vi "Optiscan_Device.vi"(7 "Device-specific in":variant, 8 "error in (no error)":errorcluster, 10 "Position in":dbl[](array[numeric]), 11 "Operation":T2(ring)) -> (0 "error out":errorcluster, 1 "Device properties":cluster{"Axes":string[], "Tolerance":dbl[][]}, 2 "Position out":dbl[](array[numeric]), 3 "Status":T1, 5 "Device-specific out":variant)   [LabVIEW 2018]
uses:
  <vilib>/Instr/_visa.llb/VISA Open Access Mode.ctl
  <vilib>/Instr/_visa.llb/VISA Configure Serial Port (Instr).vi
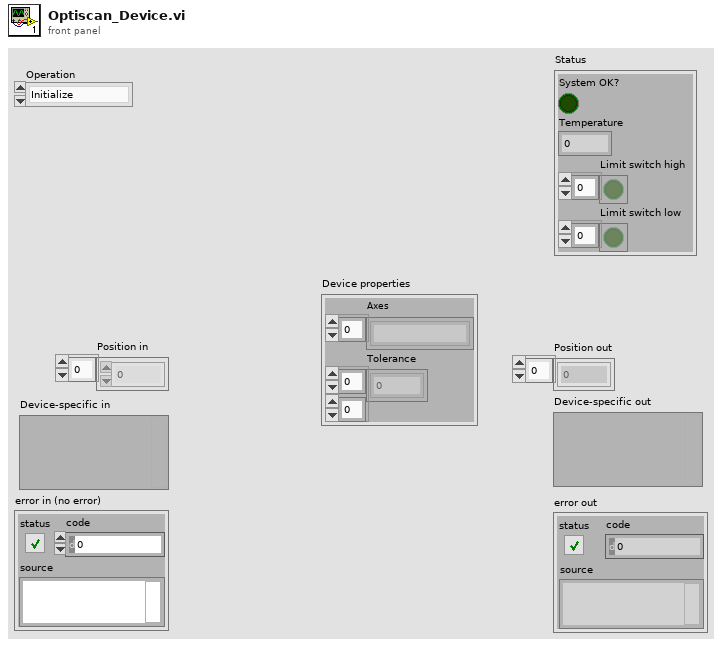
[diagram p1: front panel]
types:
  T1 = cluster{"System OK?":bool, "Temperature":dbl, "Limit switch high":bool[], "Limit switch low":bool[]}
  T2 = enum16{"Initialize", "Shut down", "Set position", "Get position", "Get status", "Other settings"}
  T3 = cluster{"COM port":refnum<visa-resource-name>, "Timeout":u32}
  T4 = typedef "VISA Open Access Mode.ctl" = u32
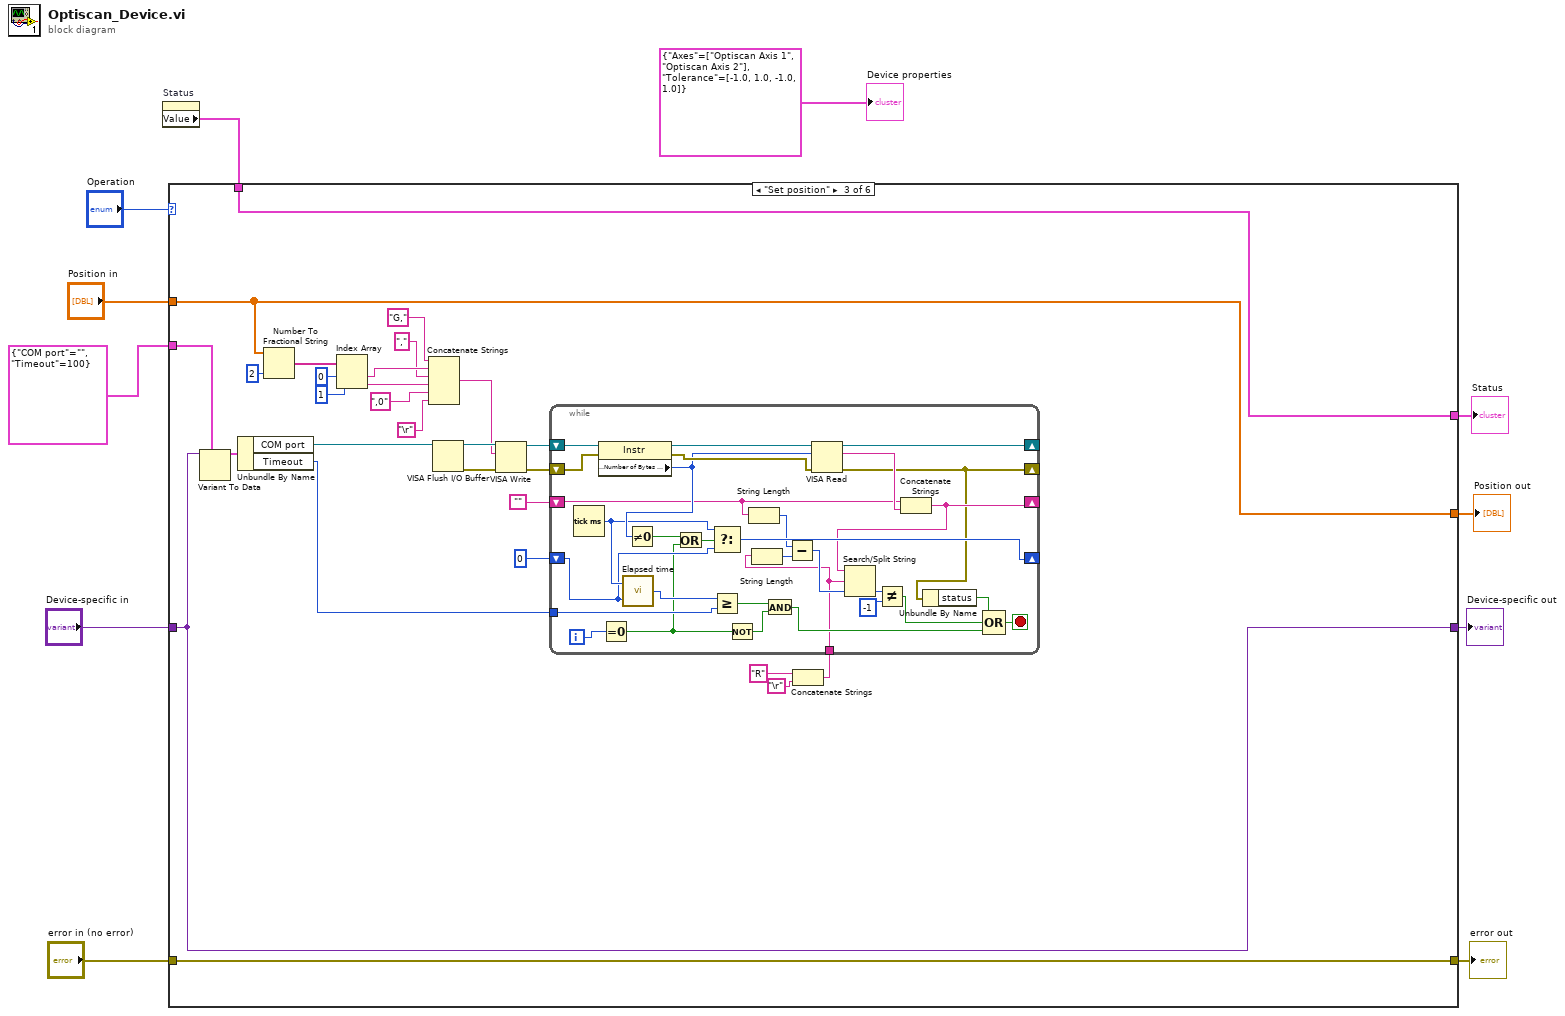
[diagram p0: block diagram]
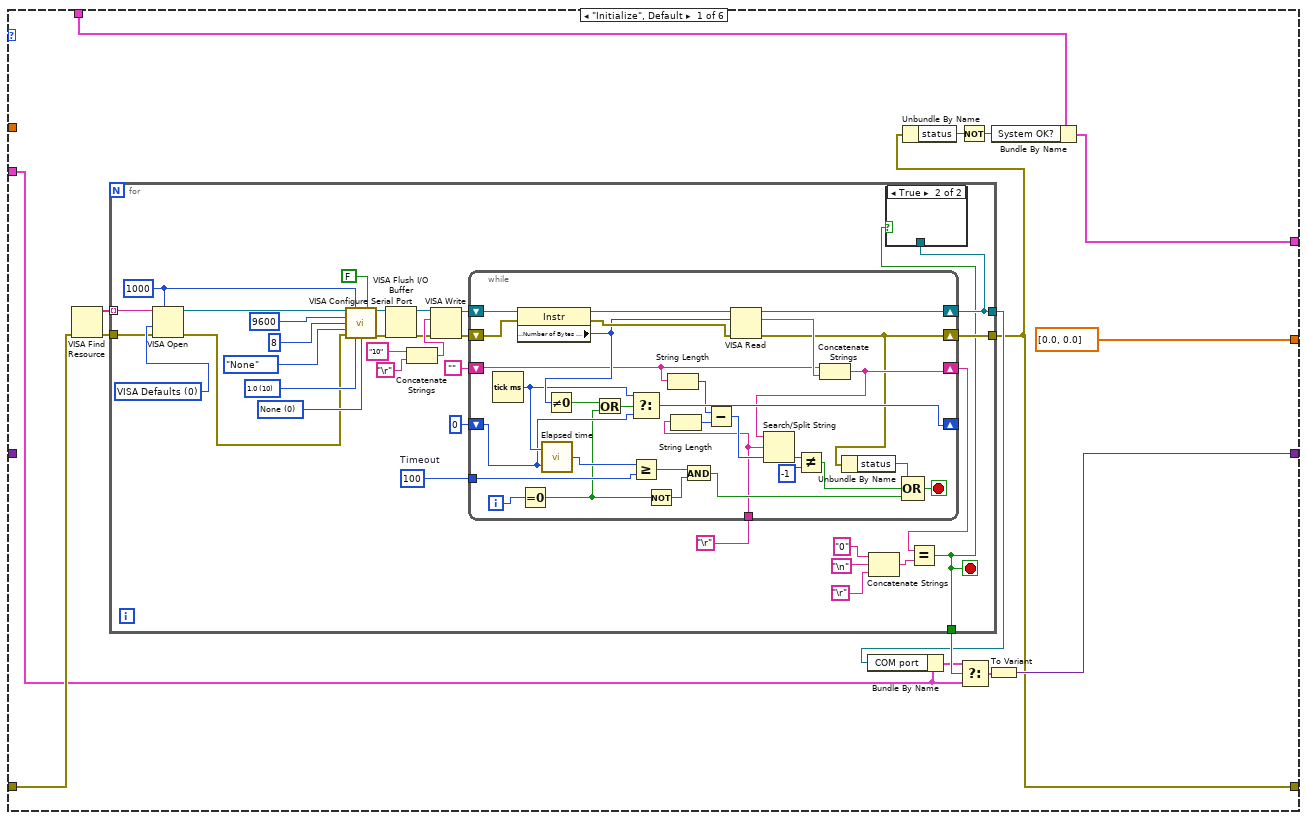
[diagram p2: hidden frame]
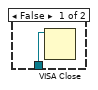
[diagram p3: hidden frame]
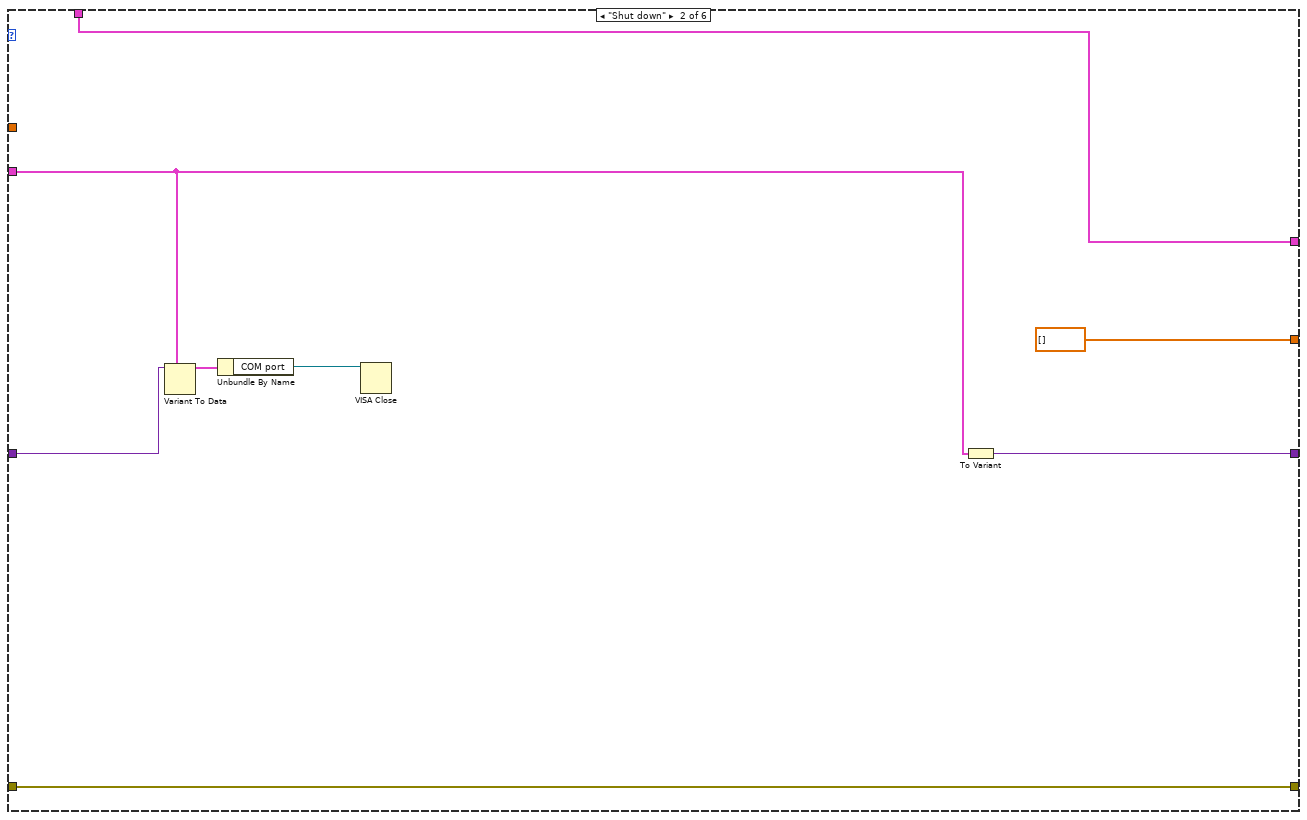
[diagram p4: hidden frame]
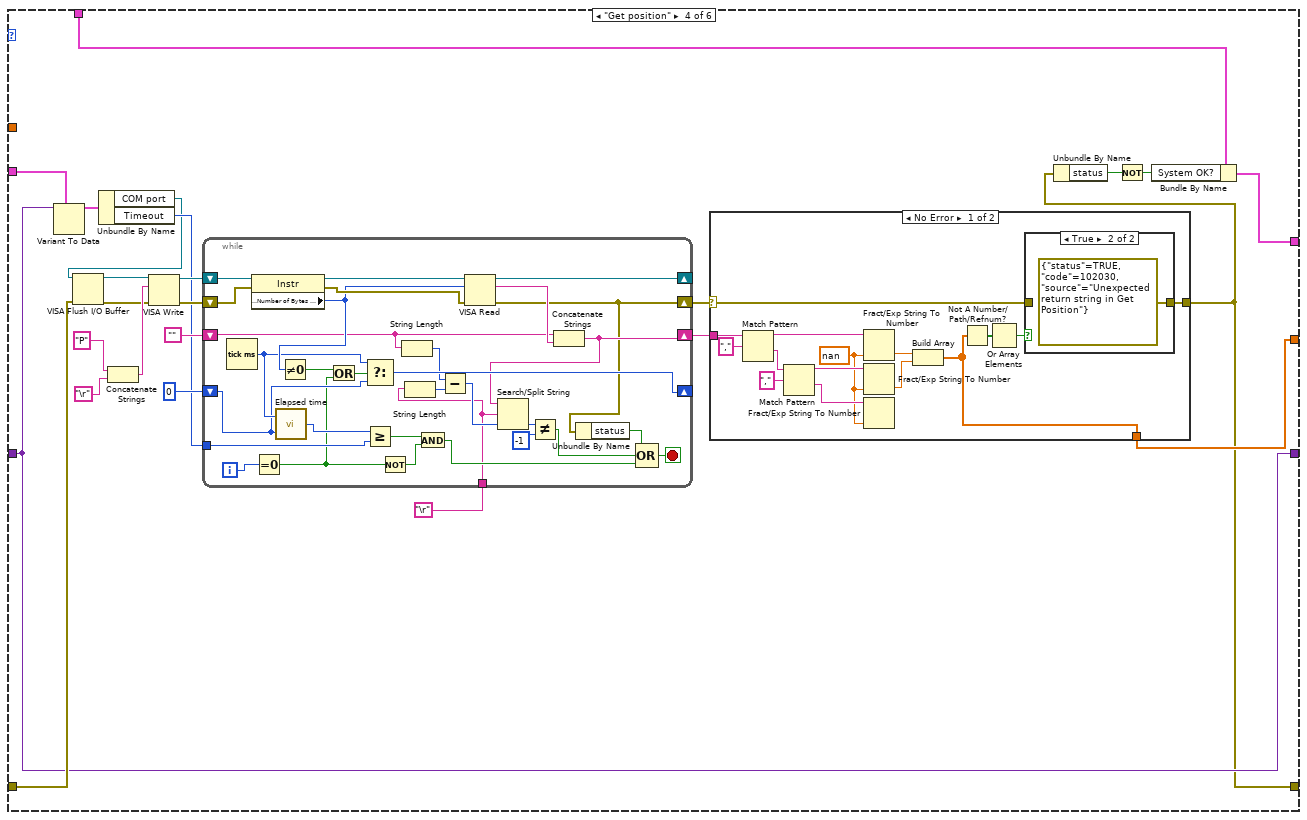
[diagram p5: hidden frame]
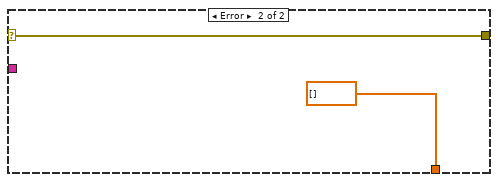
[diagram p7: hidden frame]
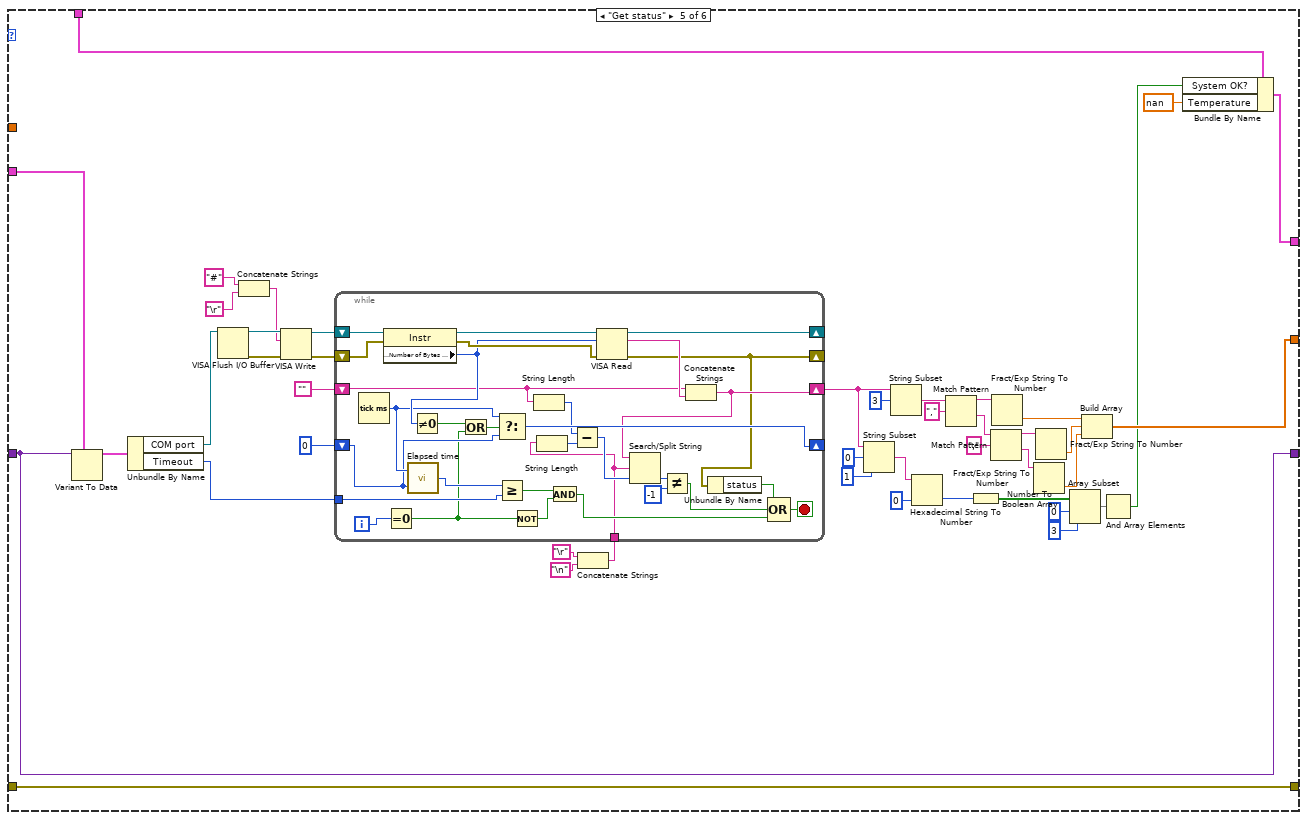
[diagram p8: hidden frame]
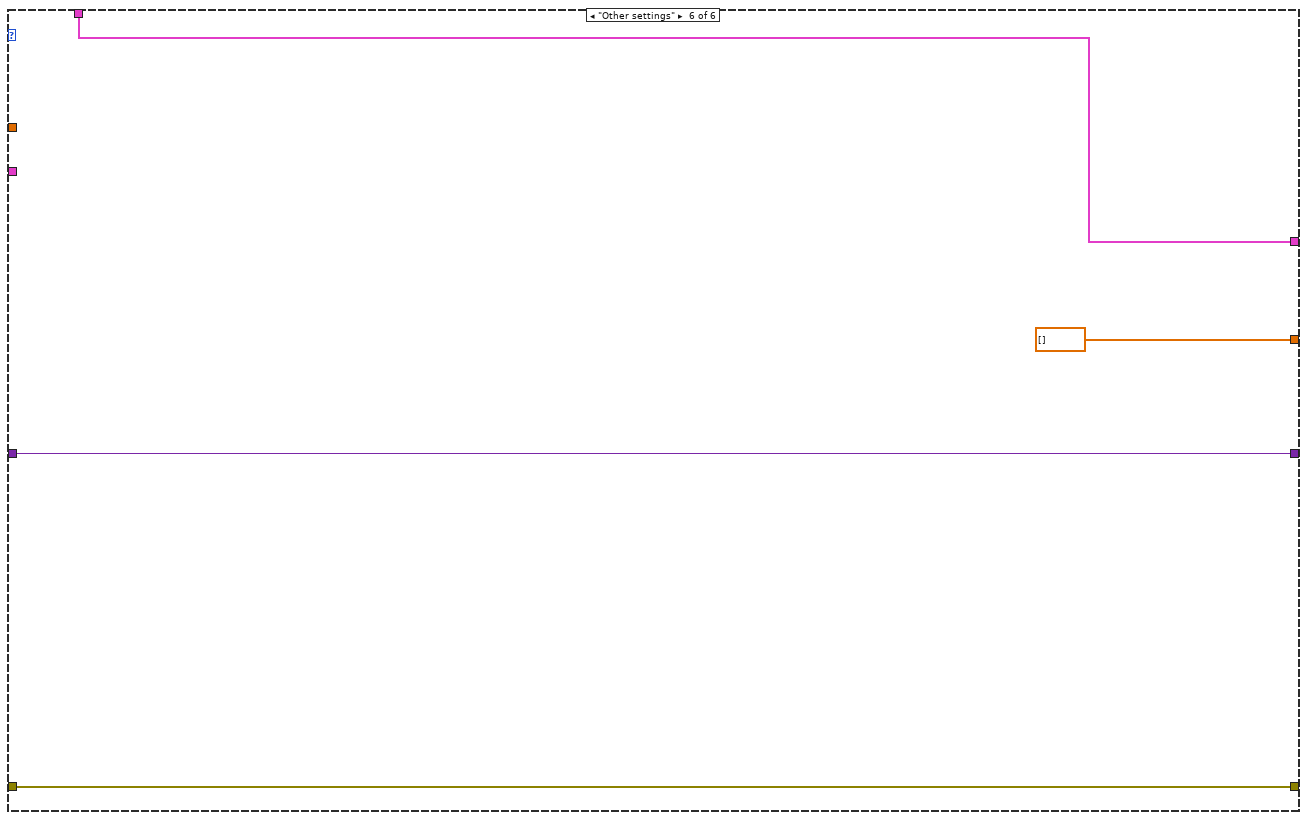
[diagram p9: hidden frame]
diagram:
  n1 = property on="Status" class="Clust (strict)"() -> ("Value"=w10:T1)  [unwired: 2 in, 2 out]
  n2 = case shown="\"Set position\"" "Operation" {
    tunnel: "Position in" -> [_ _ w101 _ _ _]
    tunnel: w10 -> [w26 w99 w127 w163 w276 w311]
    tunnel: [w25 w99 w127 w162 w275 w311] -> w9
    tunnel: "Device-specific in" -> [_ w96 w117 w170 w261 w310]
    tunnel: [dbl[] [0.0, 0.0] ("Position in") dbl[] [] ("Position in") w101 w164 w235 dbl[] [] ("Position in")] -> w6
    tunnel: [w18 w93 w117 w170 w261 w310] -> w5
    tunnel: [w15 w98 w126 w161 w273 w309] -> w4
    tunnel: "error in (no error)" -> [w16 w98 w126 w171 w273 w309]
    tunnel: T3 {"COM port"="", "Timeout"=100} -> [w13 w94 w116 w169 w260 _]
    frame "Initialize", Default {
      n3 = VISA Find Resource(8:w16) -> (0:w17:errorcluster, 3:w23:string[])  [unwired: 2 in, 1 out]
      n4 = for {
        tunnel: w23 -> [w49] mode=indexing
        tunnel: [w34] -> w21
        tunnel: [w28] -> w22
        tunnel: w17 -> [w36]
        tunnel: [w35] -> w15
        stop <- w28 stop-if-true
        w39 = u32 100  # Timeout
        w50 = u32 1000 ("timeout (10sec)")
        w52 = T4 0 items=["VISA Defaults"=0, "Exclusive Lock"=1, "Load Configured Settings"=4] ("Access Mode")
        w54 = u16 0 items=["None", "XON/XOFF", "RTS/CTS", "XON/XOFF & RTS/CTS", "DTR/DSR", "XON/XOFF & DTR/DSR"] ("flow control (0:none)")
        w55 = u16 10 items=["1.0"=10, "1.5"=15, "2.0"=20] ("stop bits (10: 1 bit)")
        n5 = VISA Open(timeout (0)=w50, access mode=w52, error in (no error)=w36, VISA resource name=w49) -> (VISA resource name=w53:refnum<visa-resource-name>, error out=w51:errorcluster)  [unwired: 1 in]
        n6 = call-poly "VISA Configure Serial Port"("VISA resource name"=w53, "timeout (10sec)"=w50, "Enable Termination\nChar (T)"=FALSE ("Enable Termination\nChar (T)"), "baud rate (9600)"=u32 9600, "data bits (8)"=u16 8, "parity (0:none)"=enum16{"None", "Odd", "Even", "Mark", "Space"}."None", "error in (no error)"=w51, "stop bits (10: 1 bit)"=w55, "flow control (0:none)"=w54) -> ("VISA resource name out"=w37:refnum<visa-resource-name>, "error out"=w38:errorcluster)  [unwired: 5 in]
        n7 = VISA Flush I/O Buffer(VISA resource name=w37, error in (no error)=w38) -> (VISA resource name out=w47:refnum<visa-resource-name>, error out=w45:errorcluster)  [unwired: 1 in]
        n8 = Concatenate Strings("10", "\r") -> (w46:string)
        n9 = VISA Write(VISA resource name=w47, write buffer=w46, error in (no error)=w45) -> (VISA resource name out=w44:refnum<visa-resource-name>, error out=w43:errorcluster)  [unwired: 1 out]
        n10 = while {
          shift-right: [w87] -> w34
          shift-left: w44 -> [w91]
          shift-right: [w61] -> w35
          shift-left: w43 -> [w90]
          shift-right: [w68] -> w32
          shift-left: "" -> [w67]
          shift-right: [w76] -> _
          shift-left: u32 0 -> [w73]
          tunnel: w39 -> [w74]
          tunnel: "\r" -> [w62]
          i -> [w79]
          stop <- w86 stop-if-true
          n11 = Tick Count (ms)() -> (millisecond timer value=w77:u32)
          n12 = property class="Instr"(reference=w91, error in=w90) -> (reference out=w89:refnum<visa-resource-name>, error out=w88:errorcluster, "Serial Settings:Number of Bytes at Serial Port"=w81:u32)
          n13 = Equal To 0?(x=w79) -> (x = 0?=w69:bool)
          n14 = call "Elapsed time.vi"("Start time (ms)"=w73, "Current time (ms)"=w77) -> ("Elapsed time"=w75:u32)
          n15 = Not Equal To 0?(x=w81) -> (x != 0?=w80:bool)
          n16 = Or(x=w80, y=w69) -> (x .or. y?=w78:bool)
          n17 = Select(t=w77, s=w78, f=w73) -> (s? t:f=w76:u32)
          n18 = Greater Or Equal?(x=w75, y=w74) -> (x >= y?=w71:bool)
          n19 = Not(x=w69) -> (.not. x?=w70:bool)
          n20 = String Length(string=w67) -> (length=w65:i32)
          n21 = String Length(string=w62) -> (length=w66:i32)
          n22 = And(x=w71, y=w70) -> (x .and. y?=w72:bool)
          n23 = Subtract(x=w65, y=w66) -> (x-y=w64:i32)
          n24 = VISA Read(VISA resource name=w89, byte count=w81, error in (no error)=w88) -> (VISA resource name out=w87:refnum<visa-resource-name>, read buffer=w85:string, error out=w61:errorcluster)  [unwired: 1 out]
          n25 = Concatenate Strings(w67, w85) -> (w68:string)
          n26 = Search/Split String(string=w68, search string/char (-)=w62, offset (0)=w64) -> (offset of match=w84:i32)  [unwired: 2 out]
          n27 = Not Equal?(x=w84, y=-1) -> (x != y?=w82:bool)
          n28 = Unbundle By Name(w61) -> ("status"=w63:bool)
          n29 = Compound Arithmetic op=OR(w63, w82, w72) -> (w86:bool)
        }
        n30 = Concatenate Strings("0" ("y"), "\n", "\r") -> (w31:string)
        n31 = Equal?(x=w32, y=w31) -> (x = y?=w28:bool)
        n32 = case shown="True" w28 {
          tunnel: w34 -> [w60 _]
          frame False {
            n33 = VISA Close(VISA resource name=w60) -> ()  [unwired: 1 in, 1 out]
          }
          frame True {
          }
        }
      }
      n34 = Bundle By Name(cluster=w13, "COM port"=w21) -> (w20:T3)
      n35 = Unbundle By Name(w15) -> ("status"=w14:bool)
      n36 = Not(x=w14) -> (.not. x?=w12:bool)
      n37 = Select(t=w20, s=w22, f=w13) -> (s? t:f=w19:T3)
      n38 = To Variant(anything=w19) -> (Variant=w18:variant)
      n39 = Bundle By Name(cluster=w26, "System OK?"=w12) -> (w25:T1)
    }
    frame "Shut down" {
      n40 = Variant To Data(type=w94, Variant=w96) -> (data=w95:T3)  [unwired: 1 in, 1 out]
      n41 = Unbundle By Name(w95) -> ("COM port"=w92:refnum<visa-resource-name>)
      n42 = VISA Close(VISA resource name=w92) -> ()  [unwired: 1 in, 1 out]
      n43 = To Variant(anything=w94) -> (Variant=w93:variant)
    }
    frame "Set position" {
      n44 = Variant To Data(type=w116, Variant=w117) -> (data=w115:T3)  [unwired: 1 in, 1 out]
      n45 = Unbundle By Name(w115) -> ("COM port"=w113:refnum<visa-resource-name>, "Timeout"=w114:u32)
      n46 = Number To Fractional String(number=w101, precision (6)=i16 2) -> (F-format string=w109:string[])  [unwired: 2 in]
      n47 = Index Array(array=w109, index #1=0 ("index"), index #2=1 ("index")) -> (element #1=w108:string, element #2=w104:string)
      n48 = Concatenate Strings("G,", w108, "," ("string"), w104, ",0" ("string"), "\r") -> (w100:string)
      n49 = VISA Flush I/O Buffer(VISA resource name=w113) -> (VISA resource name out=w125:refnum<visa-resource-name>, error out=w124:errorcluster)  [unwired: 2 in]
      n50 = VISA Write(VISA resource name=w125, write buffer=w100, error in (no error)=w124) -> (VISA resource name out=w123:refnum<visa-resource-name>, error out=w122:errorcluster)  [unwired: 1 out]
      n51 = Concatenate Strings("R" ("string"), "\r") -> (w118:string)
      n52 = while {
        shift-right: [w154] -> _
        shift-left: w123 -> [w158]
        shift-right: [w128] -> _
        shift-left: w122 -> [w157]
        shift-right: [w135] -> _
        shift-left: "" -> [w134]
        shift-right: [w143] -> _
        shift-left: u32 0 -> [w140]
        tunnel: w114 -> [w141]
        tunnel: w118 -> [w129]
        i -> [w146]
        stop <- w153 stop-if-true
        n53 = Tick Count (ms)() -> (millisecond timer value=w144:u32)
        n54 = property class="Instr"(reference=w158, error in=w157) -> (reference out=w156:refnum<visa-resource-name>, error out=w155:errorcluster, "Serial Settings:Number of Bytes at Serial Port"=w148:u32)
        n55 = Equal To 0?(x=w146) -> (x = 0?=w136:bool)
        n56 = call "Elapsed time.vi"("Start time (ms)"=w140, "Current time (ms)"=w144) -> ("Elapsed time"=w142:u32)
        n57 = Not Equal To 0?(x=w148) -> (x != 0?=w147:bool)
        n58 = Or(x=w147, y=w136) -> (x .or. y?=w145:bool)
        n59 = Select(t=w144, s=w145, f=w140) -> (s? t:f=w143:u32)
        n60 = Greater Or Equal?(x=w142, y=w141) -> (x >= y?=w138:bool)
        n61 = Not(x=w136) -> (.not. x?=w137:bool)
        n62 = String Length(string=w134) -> (length=w132:i32)
        n63 = String Length(string=w129) -> (length=w133:i32)
        n64 = And(x=w138, y=w137) -> (x .and. y?=w139:bool)
        n65 = Subtract(x=w132, y=w133) -> (x-y=w131:i32)
        n66 = VISA Read(VISA resource name=w156, byte count=w148, error in (no error)=w155) -> (VISA resource name out=w154:refnum<visa-resource-name>, read buffer=w152:string, error out=w128:errorcluster)  [unwired: 1 out]
        n67 = Concatenate Strings(w134, w152) -> (w135:string)
        n68 = Search/Split String(string=w135, search string/char (-)=w129, offset (0)=w131) -> (offset of match=w151:i32)  [unwired: 2 out]
        n69 = Not Equal?(x=w151, y=-1) -> (x != y?=w149:bool)
        n70 = Unbundle By Name(w128) -> ("status"=w130:bool)
        n71 = Compound Arithmetic op=OR(w130, w149, w139) -> (w153:bool)
      }
    }
    frame "Get position" {
      n72 = Variant To Data(type=w169, Variant=w170) -> (data=w168:T3)  [unwired: 1 in, 1 out]
      n73 = Unbundle By Name(w168) -> ("COM port"=w166:refnum<visa-resource-name>, "Timeout"=w167:u32)
      n74 = VISA Flush I/O Buffer(VISA resource name=w166, error in (no error)=w171) -> (VISA resource name out=w181:refnum<visa-resource-name>, error out=w179:errorcluster)  [unwired: 1 in]
      n75 = Concatenate Strings("P", "\r") -> (w180:string)
      n76 = VISA Write(VISA resource name=w181, write buffer=w180, error in (no error)=w179) -> (VISA resource name out=w178:refnum<visa-resource-name>, error out=w177:errorcluster)  [unwired: 1 out]
      n77 = while {
        shift-right: [w228] -> _
        shift-left: w178 -> [w232]
        shift-right: [w202] -> w172
        shift-left: w177 -> [w231]
        shift-right: [w209] -> w173
        shift-left: "" -> [w208]
        shift-right: [w217] -> _
        shift-left: u32 0 -> [w214]
        tunnel: w167 -> [w215]
        tunnel: "\r" -> [w203]
        i -> [w220]
        stop <- w227 stop-if-true
        n78 = Tick Count (ms)() -> (millisecond timer value=w218:u32)
        n79 = property class="Instr"(reference=w232, error in=w231) -> (reference out=w230:refnum<visa-resource-name>, error out=w229:errorcluster, "Serial Settings:Number of Bytes at Serial Port"=w222:u32)
        n80 = Equal To 0?(x=w220) -> (x = 0?=w210:bool)
        n81 = call "Elapsed time.vi"("Start time (ms)"=w214, "Current time (ms)"=w218) -> ("Elapsed time"=w216:u32)
        n82 = Not Equal To 0?(x=w222) -> (x != 0?=w221:bool)
        n83 = Or(x=w221, y=w210) -> (x .or. y?=w219:bool)
        n84 = Select(t=w218, s=w219, f=w214) -> (s? t:f=w217:u32)
        n85 = Greater Or Equal?(x=w216, y=w215) -> (x >= y?=w212:bool)
        n86 = Not(x=w210) -> (.not. x?=w211:bool)
        n87 = String Length(string=w208) -> (length=w206:i32)
        n88 = String Length(string=w203) -> (length=w207:i32)
        n89 = And(x=w212, y=w211) -> (x .and. y?=w213:bool)
        n90 = Subtract(x=w206, y=w207) -> (x-y=w205:i32)
        n91 = VISA Read(VISA resource name=w230, byte count=w222, error in (no error)=w229) -> (VISA resource name out=w228:refnum<visa-resource-name>, read buffer=w226:string, error out=w202:errorcluster)  [unwired: 1 out]
        n92 = Concatenate Strings(w208, w226) -> (w209:string)
        n93 = Search/Split String(string=w209, search string/char (-)=w203, offset (0)=w205) -> (offset of match=w225:i32)  [unwired: 2 out]
        n94 = Not Equal?(x=w225, y=-1) -> (x != y?=w223:bool)
        n95 = Unbundle By Name(w202) -> ("status"=w204:bool)
        n96 = Compound Arithmetic op=OR(w204, w223, w213) -> (w227:bool)
      }
      n97 = case shown="No Error" w172 {
        selector: w172 -> [w196 w201]
        tunnel: w173 -> [w186 _]
        tunnel: [w197 w201] -> w161
        tunnel: [w185 dbl[] []] -> w164
        frame No Error {
          w183 = nan ("default (0 DBL)")
          n98 = Match Pattern(string=w186, regular expression=",") -> (before substring=w192:string, after substring=w190:string)  [unwired: 1 in, 2 out]
          n99 = Match Pattern(string=w190, regular expression=",") -> (before substring=w189:string, after substring=w188:string)  [unwired: 1 in, 2 out]
          n100 = Fract/Exp String To Number(string=w192, default (0 dbl)=w183) -> (number=w193:dbl)  [unwired: 2 in, 1 out]
          n101 = Fract/Exp String To Number(string=w189, default (0 dbl)=w183) -> (number=w187:dbl)  [unwired: 2 in, 1 out]
          n102 = Fract/Exp String To Number(string=w188, default (0 dbl)=w183) -> ()  [unwired: 2 in, 2 out]
          n103 = Build Array(w193, w187) -> (w185:dbl[])
          n104 = Not A Number/Path/Refnum?(number/path/refnum=w185) -> (NaN/Path/Refnum?=w195:bool[])
          n105 = Or Array Elements(Boolean array=w195) -> (logical OR=w184:bool)
          n106 = case shown="True" w184 {
            tunnel: [w198 errorcluster {"status"=TRUE, "code"=102030, "source"="Unexpected return string in Get Position"} ("error IO")] -> w197
            tunnel: w196 -> [w198 _]
            frame False {
            }
            frame True {
            }
          }
        }
        frame Error {
        }
      }
      n107 = Unbundle By Name(w161) -> ("status"=w160:bool)
      n108 = Not(x=w160) -> (.not. x?=w159:bool)
      n109 = Bundle By Name(cluster=w163, "System OK?"=w159) -> (w162:T1)
    }
    frame "Get status" {
      n110 = Variant To Data(type=w260, Variant=w261) -> (data=w259:T3)  [unwired: 1 in, 1 out]
      n111 = Unbundle By Name(w259) -> ("COM port"=w257:refnum<visa-resource-name>, "Timeout"=w258:u32)
      n112 = VISA Flush I/O Buffer(VISA resource name=w257) -> (VISA resource name out=w272:refnum<visa-resource-name>, error out=w271:errorcluster)  [unwired: 2 in]
      n113 = Concatenate Strings("#", "\r") -> (w262:string)
      n114 = VISA Write(VISA resource name=w272, write buffer=w262, error in (no error)=w271) -> (VISA resource name out=w270:refnum<visa-resource-name>, error out=w269:errorcluster)  [unwired: 1 out]
      n115 = Concatenate Strings("\r", "\n") -> (w264:string)
      n116 = while {
        shift-right: [w303] -> _
        shift-left: w270 -> [w307]
        shift-right: [w277] -> _
        shift-left: w269 -> [w306]
        shift-right: [w284] -> w236
        shift-left: "" -> [w283]
        shift-right: [w292] -> _
        shift-left: u32 0 -> [w289]
        tunnel: w258 -> [w290]
        tunnel: w264 -> [w278]
        i -> [w295]
        stop <- w302 stop-if-true
        n117 = Tick Count (ms)() -> (millisecond timer value=w293:u32)
        n118 = property class="Instr"(reference=w307, error in=w306) -> (reference out=w305:refnum<visa-resource-name>, error out=w304:errorcluster, "Serial Settings:Number of Bytes at Serial Port"=w297:u32)
        n119 = Equal To 0?(x=w295) -> (x = 0?=w285:bool)
        n120 = call "Elapsed time.vi"("Start time (ms)"=w289, "Current time (ms)"=w293) -> ("Elapsed time"=w291:u32)
        n121 = Not Equal To 0?(x=w297) -> (x != 0?=w296:bool)
        n122 = Or(x=w296, y=w285) -> (x .or. y?=w294:bool)
        n123 = Select(t=w293, s=w294, f=w289) -> (s? t:f=w292:u32)
        n124 = Greater Or Equal?(x=w291, y=w290) -> (x >= y?=w287:bool)
        n125 = Not(x=w285) -> (.not. x?=w286:bool)
        n126 = String Length(string=w283) -> (length=w281:i32)
        n127 = String Length(string=w278) -> (length=w282:i32)
        n128 = And(x=w287, y=w286) -> (x .and. y?=w288:bool)
        n129 = Subtract(x=w281, y=w282) -> (x-y=w280:i32)
        n130 = VISA Read(VISA resource name=w305, byte count=w297, error in (no error)=w304) -> (VISA resource name out=w303:refnum<visa-resource-name>, read buffer=w301:string, error out=w277:errorcluster)  [unwired: 1 out]
        n131 = Concatenate Strings(w283, w301) -> (w284:string)
        n132 = Search/Split String(string=w284, search string/char (-)=w278, offset (0)=w280) -> (offset of match=w300:i32)  [unwired: 2 out]
        n133 = Not Equal?(x=w300, y=-1) -> (x != y?=w298:bool)
        n134 = Unbundle By Name(w277) -> ("status"=w279:bool)
        n135 = Compound Arithmetic op=OR(w279, w298, w288) -> (w302:bool)
      }
      n136 = String Subset(string=w236, offset (0)=0, length (rest)=1 ("length (rest)")) -> (substring=w253:string)
      n137 = String Subset(string=w236, offset (0)=3) -> (substring=w241:string)  [unwired: 1 in]
      n138 = Hexadecimal String To Number(string=w253, default (0uL)=u16 0 ("default (0 U32)")) -> (number=w251:u16)  [unwired: 1 in, 1 out]
      n139 = Match Pattern(string=w241, regular expression=",") -> (before substring=w248:string, after substring=w246:string)  [unwired: 1 in, 2 out]
      n140 = Number To Boolean Array(number=w251) -> (Boolean array=w239:bool[])
      n141 = Match Pattern(string=w246, regular expression=",") -> (before substring=w245:string, after substring=w244:string)  [unwired: 1 in, 2 out]
      n142 = Fract/Exp String To Number(string=w248) -> (number=w249:dbl)  [unwired: 3 in, 1 out]
      n143 = Fract/Exp String To Number(string=w244) -> (number=w242:dbl)  [unwired: 3 in, 1 out]
      n144 = Fract/Exp String To Number(string=w245) -> (number=w243:dbl)  [unwired: 3 in, 1 out]
      n145 = Array Subset(array=w239, index=0, length=3) -> (w234:bool[])
      n146 = Build Array(w249, w243, w242) -> (w235:dbl[])
      n147 = And Array Elements(Boolean array=w234) -> (logical AND=w233:bool)
      n148 = Bundle By Name(cluster=w276, "System OK?"=w233, "Temperature"=nan) -> (w275:T1)
    }
    frame "Other settings" {
    }
  }
  "Status" <- w9
  "Device-specific out" <- w5
  "error out" <- w4
  "Position out" <- w6
  "Device properties" <- cluster{"Axes":string[], "Tolerance":dbl[][]} {"Axes"=["Optiscan Axis 1", "Optiscan Axis 2"], "Tolerance"=[[-1.0, 1.0], [-1.0, 1.0]]} ("Device properties")
